vi "SeguidordeVueltas.vi"() -> ()   [LabVIEW 2011]
panel:
  out "Gauge":dbl(knob) scale=0.0..360.0
  in  "stop":bool
  out "Diagrama Fasorial":picture
  out "floor(x/y)":i32
  out "x-y*floor(x/y)":i32
  in  "y":i32
  out "Numeric":i32
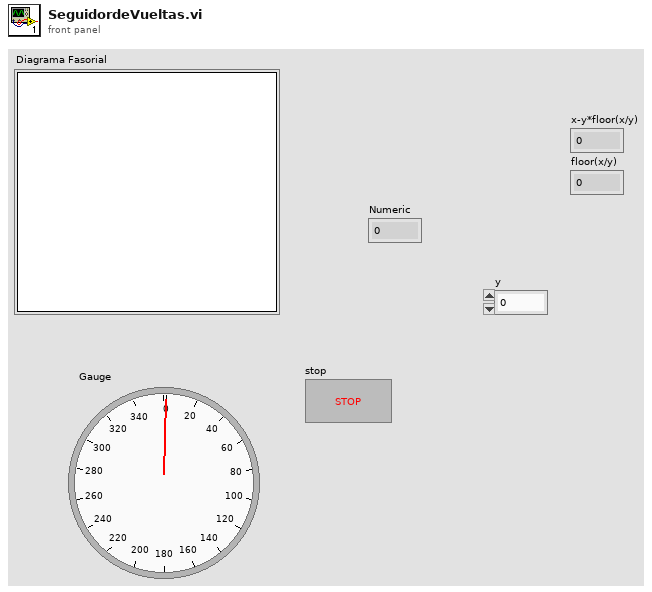
[diagram p1: front panel]
types:
  T1 = typedef "LVBoundsTypeDef.ctl" = cluster{"Width":u32, "Height":u32}
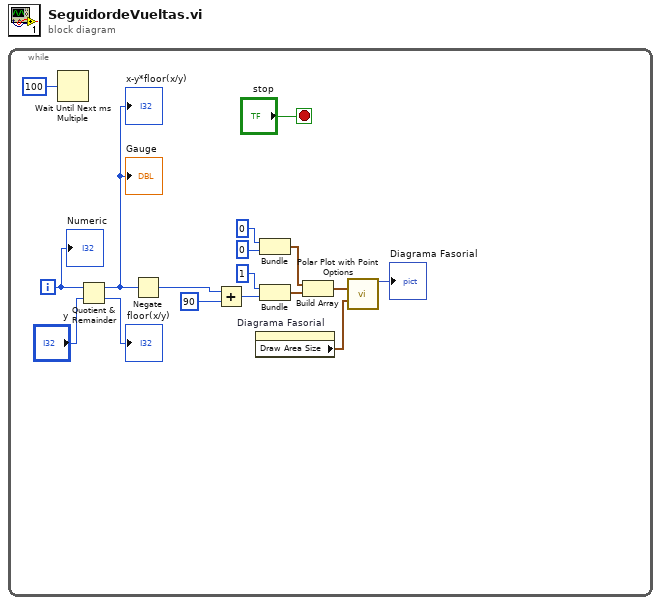
[diagram p0: block diagram]
diagram:
  n1 = while {
    i -> [w17]
    stop <- "stop" stop-if-true
    n2 = Wait Until Next ms Multiple(millisecond multiple=u32 100) -> ()  [unwired: 1 out]
    n3 = Quotient & Remainder(x=w17, y="y") -> (x-y*floor(x/y)=w4:i32, floor(x/y)=→"floor(x/y)":i32)
    "x-y*floor(x/y)" <- w4
    "Gauge" <- w4
    n4 = Negate(x=w4) -> (-x=w2:i32)
    n5 = Add(x=w2, y=90) -> (x+y=w1:i32)
    n6 = property on="Diagrama Fasorial" class="Pict"() -> ("Draw Area Size"=w13:T1)  [unwired: 2 in, 2 out]
    n7 = Bundle(0, 0) -> (w10:cluster{i32, i32})  [unwired: 1 in]
    n8 = Bundle(1, w1) -> (w7:cluster{i32, i32})  [unwired: 1 in]
    n9 = Build Array(w10, w7) -> (w9:cluster{i32, i32}[])
    n10 = call <vilib>:"Polar Plot with Point Options.vi"("data array [mag, phase (deg)]"=w9, "dimensions (w,h)"=w13) -> ("new picture"=→"Diagrama Fasorial":picture)  [unwired: 13 in]
    "Numeric" <- w17
  }
